vi "Stop Core.vi"(10 "final error code":i32, 11 "CS++GoBangServer in":refnum<class "CS++GoBangServer.lvclass">) -> (3 "CS++GoBangServer out":refnum<class "CS++GoBangServer.lvclass">)   [LabVIEW 2014, in "GoBang.lvlib" / "CS++GoBangServer.lvclass"]
doc: "(<B>Filename</B>: Actor Framework.lvlib:Actor.lvclass:Stop Core.vi)\n\nDefines what the actor does before it stops. Use the <B>final error code</B> input to determine whether the actor shut down in response to an error.\n\nBy default, this method does nothing. A descendant class may override it to define behavior, such as shutting down any processes the actor initiated in its override of the Actor Core method."
uses:
  CS++GoBangServer.lvclass
  CS++GoBangServer.lvclass/CS++GoBangServer.ctl
  <vilib>/ActorFramework/Message Enqueuer/Message Enqueuer.lvclass/Message Enqueuer.ctl
  <vilib>/ActorFramework/Message Enqueuer/Enqueue.vi
  <vilib>/ActorFramework/Message Priority Queue/Priority Enqueue.vi
  <vilib>/ActorFramework/Actor/Actor.lvclass
  <vilib>/ActorFramework/Stop Msg/Stop Msg.lvclass
  <vilib>/NI/Actors/Linked Network Actor/Linked Network Actor Messages/Disconnect Msg/Disconnect Msg.lvclass
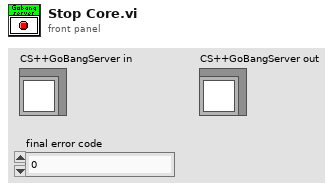
[diagram p1: front panel]
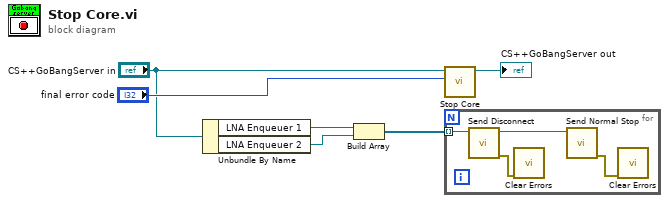
[diagram p0: block diagram]
diagram:
  n1 = Unbundle By Name("CS++GoBangServer in") -> ("LNA Enqueuer 1"=w3:refnum<class "Message Enqueuer.lvclass">, "LNA Enqueuer 2"=w2:refnum<class "Message Enqueuer.lvclass">)
  n2 = Build Array(w3, w2) -> (w1:refnum<class "Message Enqueuer.lvclass">[])
  n3 = call-parent "Stop Core.vi"("final error code"="final error code", "Actor in"="CS++GoBangServer in") -> ("Actor out"=→"CS++GoBangServer out":refnum<class "CS++GoBangServer.lvclass">)  [unwired: 9 in]
  n4 = for {
    tunnel: w1 -> [w7] mode=indexing
    n5 = call <vilib>:"Send Disconnect.vi"("Message Enqueuer"=w7) -> ("error out"=w9:errorcluster, "Message Enqueuer out"=w10:refnum<class "Message Enqueuer.lvclass">)  [unwired: 9 in]
    n6 = call <vilib>:"Clear Errors.vi"("error in (no error)"=w9) -> ()  [unwired: 5 in, 2 out]
    n7 = call <vilib>:"Send Normal Stop.vi"("Message Enqueuer"=w10) -> ("error out"=w8:errorcluster)  [unwired: 10 in]
    n8 = call <vilib>:"Clear Errors.vi"("error in (no error)"=w8) -> ()  [unwired: 5 in, 2 out]
  }
